vi "Ring Value to String.vi"(10 "Value":i32, 11 "Ring in":refnum<vi>) -> (3 "String":string)   [LabVIEW 2021]
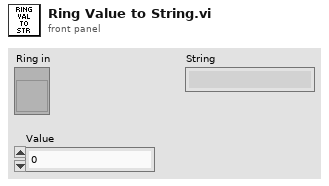
[diagram p1: front panel]
types:
  T1 = typedef "LVStringsAndValuesArrayTypeDef_I32.ctl" = cluster{"String":string, "Value":i32}[]
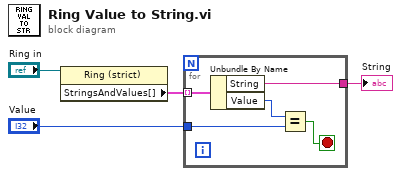
[diagram p0: block diagram]
diagram:
  n1 = property on="Property Node" class="Ring (strict)"(reference="Ring in") -> ("StringsAndValues[]"=w3:T1)  [unwired: 1 in, 2 out]
  n2 = for {
    tunnel: "Value" -> [w8]
    tunnel: [w7] -> w4
    tunnel: w3 -> [w6] mode=indexing
    stop <- w5 stop-if-true
    n3 = Unbundle By Name(w6) -> ("String"=w7:string, "Value"=w9:i32)
    n4 = Equal?(x=w9, y=w8) -> (x = y?=w5:bool)
  }
  "String" <- w4
